vi "ddsAmpArrayConvert.vi"(7 "Pre 3.0 AOM driver version?":bool, 10 "Register":dbl=3.0 min=0.0 max=15.0 step=1.0 format="%#.6f", 11 "Amplitude Array (0-1)":dbl[](array[numeric])=[0.49999872] min=0.0 max=1.0 step=6.1035e-05 format="%.4g") -> (3 "Characters for FPGA":string="L31???\r\n")   [LabVIEW 2013, in "DDS9954_v2013.lvlib"]
uses:
  DDS9954_v2013.lvlib
  dataToAscii_16bit.vi
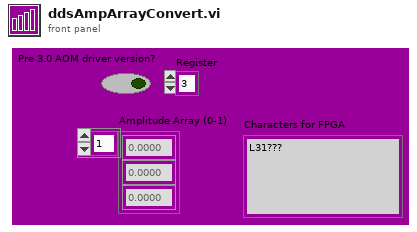
[diagram p1: front panel]
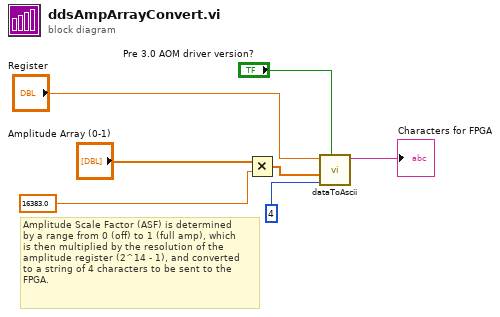
[diagram p0: block diagram]
diagram:
  # "Amplitude Scale Factor (ASF) is determined\nby a range from 0 (off) to 1 (full amp), which\nis then multiplied by the resolution of the\namplitude register (2^14 - 1), and converted\nto a string of 4 characters to be sent to the \nFPGA."
  n1 = Multiply(x="Amplitude Array (0-1)", y=16383.0) -> (x*y=w3:dbl[])
  n2 = call-poly "dataToAscii.vi"("Pre 3.0 AOM driver version?"="Pre 3.0 AOM driver version?", "HEX min width (pre 3.0)"=u8 4, "Input Data"=w3, "Register"="Register") -> ("Characters to FPGA"=→"Characters for FPGA":string)  [unwired: 7 in]
